vi "Administer Tables UI.vi"() -> ()   [LabVIEW 2019, in "LV-Data.PGSQL.lvclass"]
uses:
  LV-Data.PGSQL.lvclass
  Typedefs/Datatypes--enum.ctl
  <userlib>/_OpenG.lib/array/array.llb/Search 1D Array (String)__ogtk.vi
panel:
  in  "Safety":bool=TRUE
  in  "Delete Selected Table":bool
  in  "Delete Selected Column":bool
  in  "Rename Selected Table":bool
  in  "Update Selected Column Units":bool
  in  "Rename Selected Column":bool
  out "Path":string="llab_038:d001(TEST_TABLE--new_stuff(hippos))"
  out "selected table":string
  in  "New Column Units":string="discoveries"
  in  "New Column Name":string="successfulness"
  in  "Create New Column":bool
  in  "New Column Type":T1
  in  "Columns":i32(listbox)=-1
  in  "New Table Name":string="TEST_TABLE_2"
  in  "Create New Table":bool
  in  "Tables":i32(listbox)=-1
  in  "STOP":bool
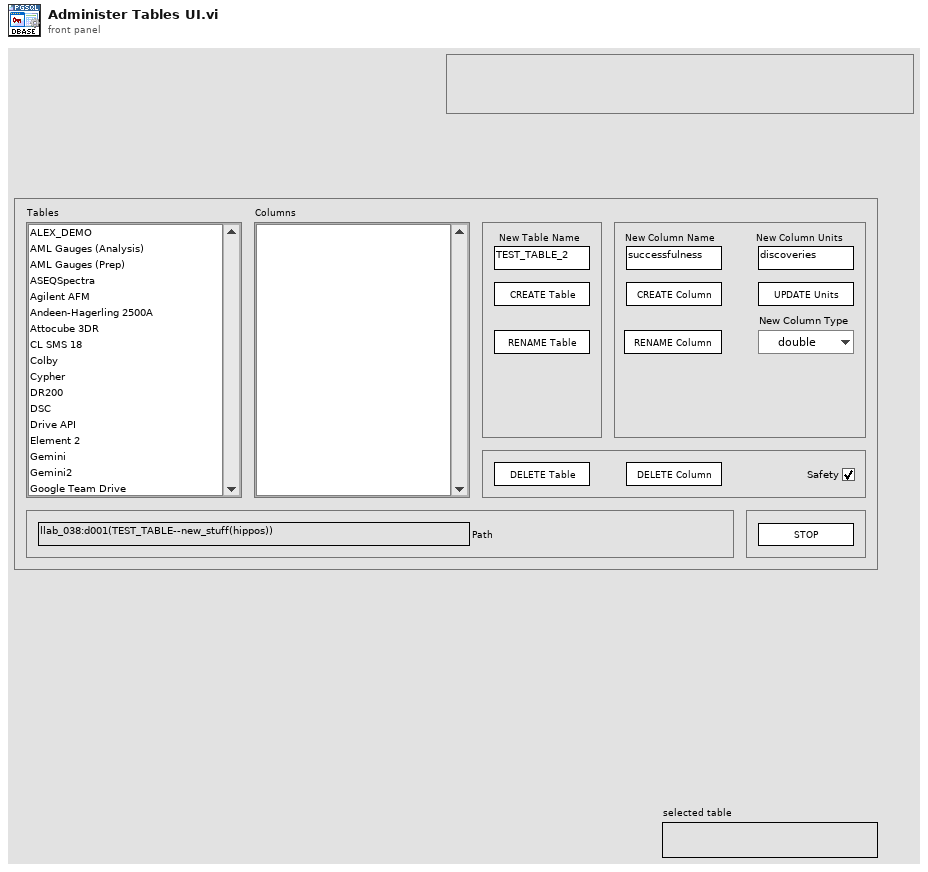
[diagram p1: front panel]
types:
  T1 = typedef "LV-Data.PGSQL.lvclass/Datatypes--enum.ctl" = enum16{"double", "string", "json", "integer", "boolean"}
  T2 = enum32{"Invalid", "Standard", "Closed", "Hidden", "Minimized", "Maximized"}
  T3 = enum32{"invalid app kind", "Development System", "Run Time System", "Student Edition", "Embedded LabVIEW", "Evaluation", "Custom"}
  T4 = cluster{"Core":cluster{"Current VI Reference":refnum<vi>, "Close Panel on Exit?":bool}, "Data.PG":refnum<class "LV-Data.PGSQL.lvclass">, "table names":string[], "table paths":string[], "column names":string[], "column units":string[], "column paths":string[], "new table name":string, "new column name":string, "new column data type":T1, "new column units":string, "selected table":string, "selected column":string, "selected table path":string, "selected column path":string, "selected column units":string}
  T5 = cluster{"Current VI Reference":refnum<vi>, "Close Panel on Exit?":bool}
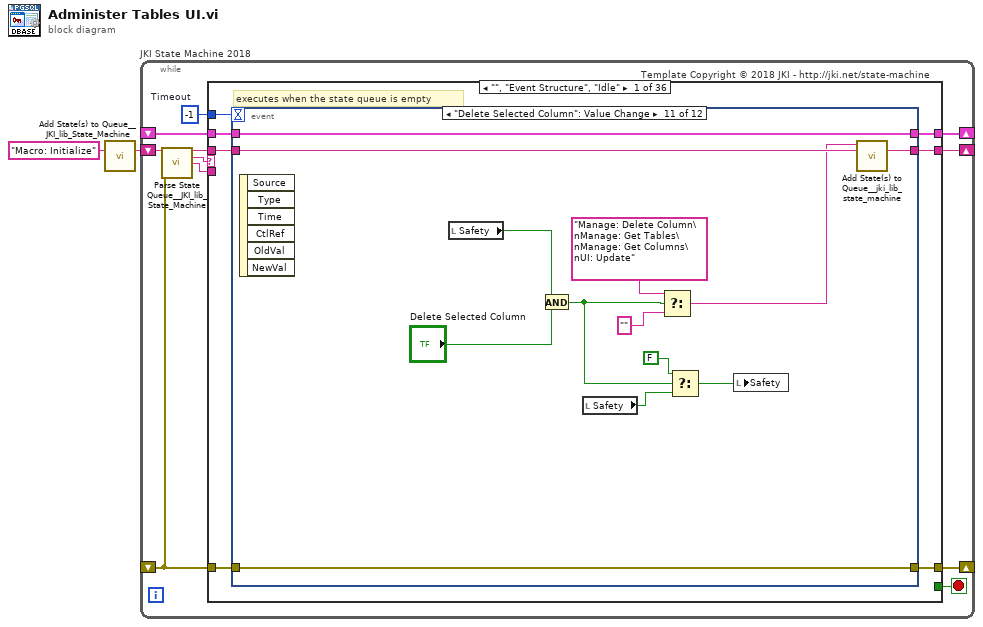
[diagram p0: block diagram]
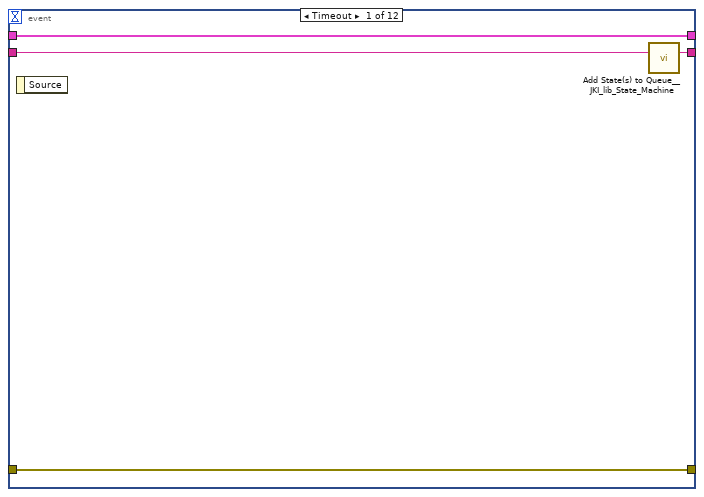
[diagram p2: hidden frame]
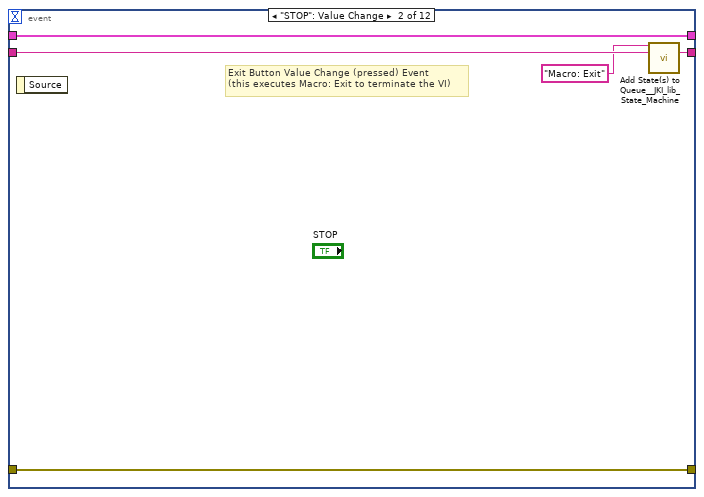
[diagram p3: hidden frame]
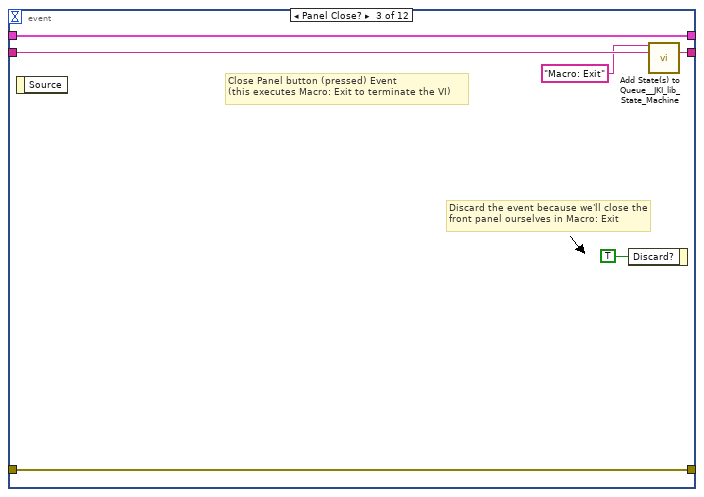
[diagram p4: hidden frame]
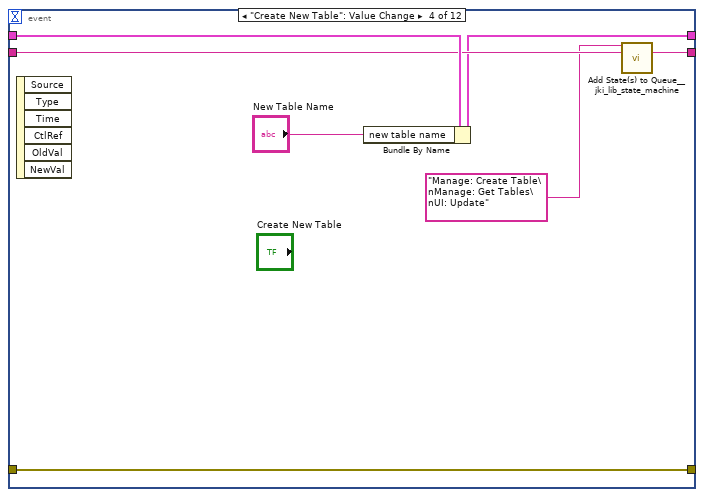
[diagram p5: hidden frame]
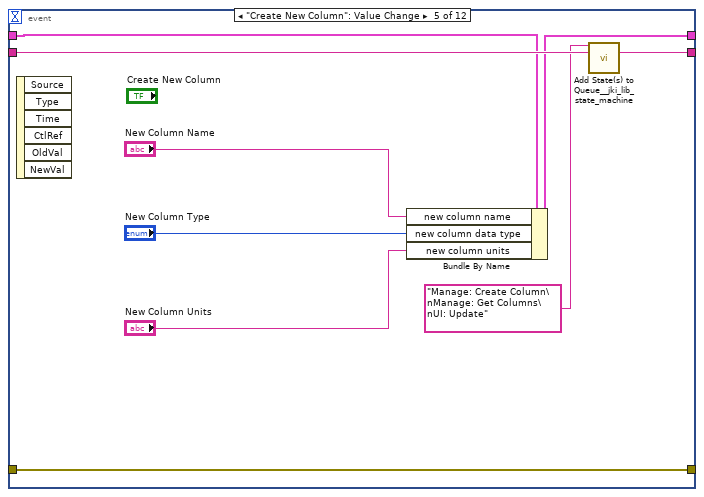
[diagram p6: hidden frame]
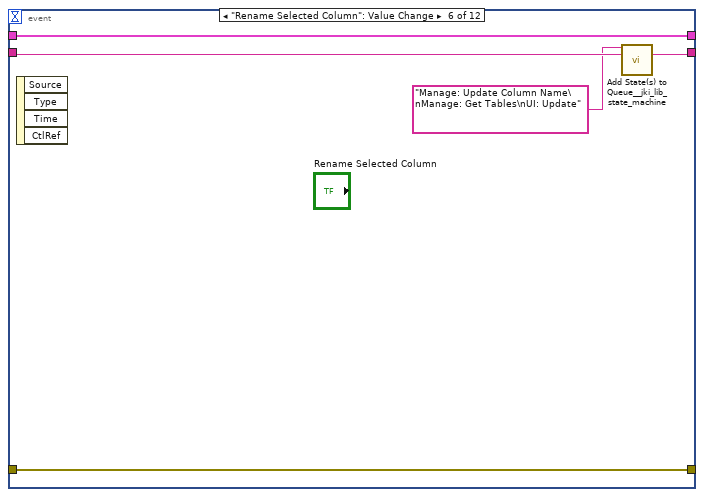
[diagram p7: hidden frame]
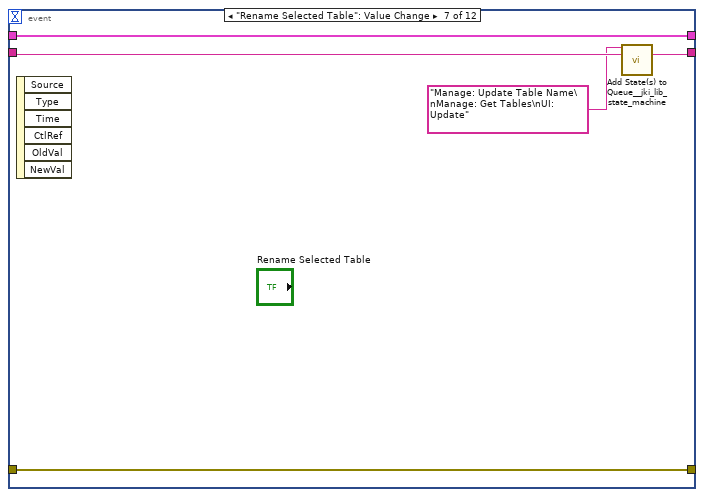
[diagram p8: hidden frame]
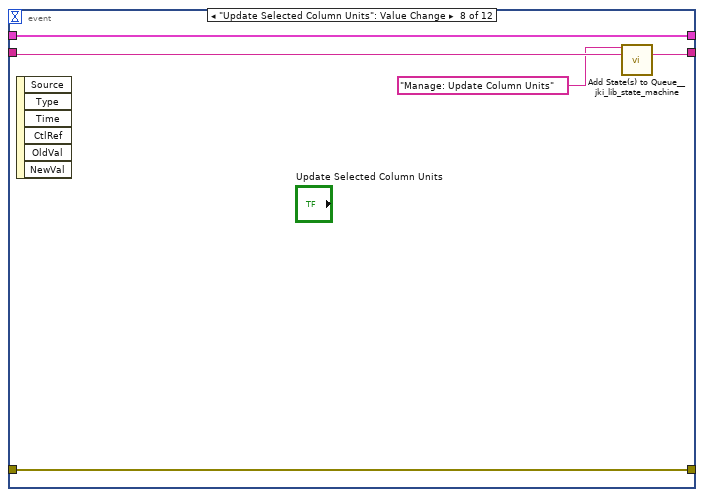
[diagram p9: hidden frame]
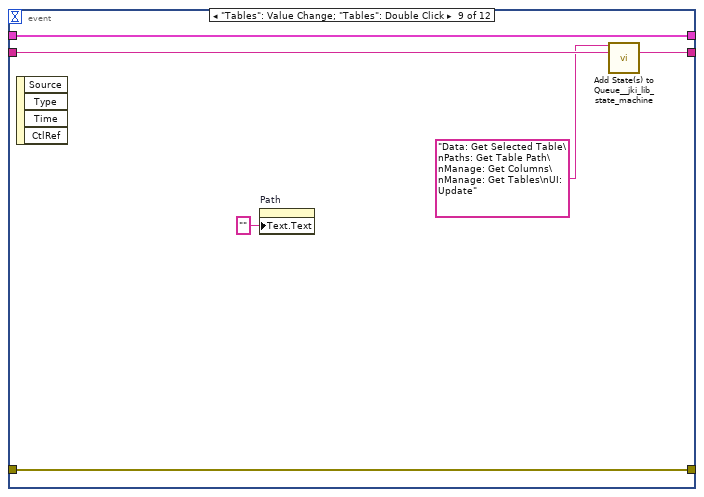
[diagram p10: hidden frame]
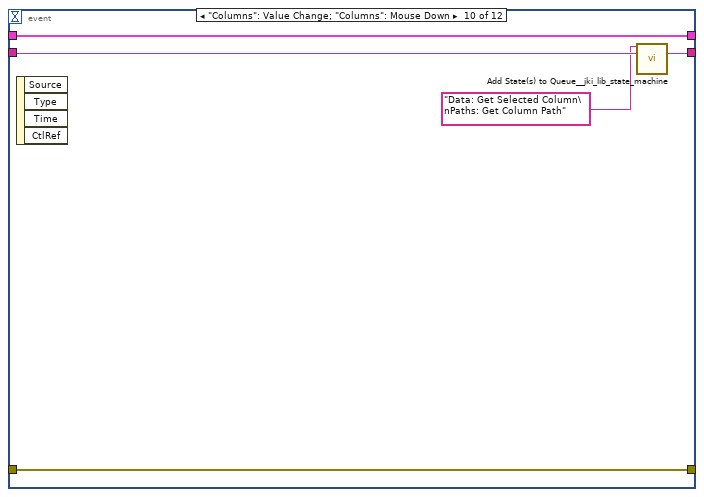
[diagram p11: hidden frame]
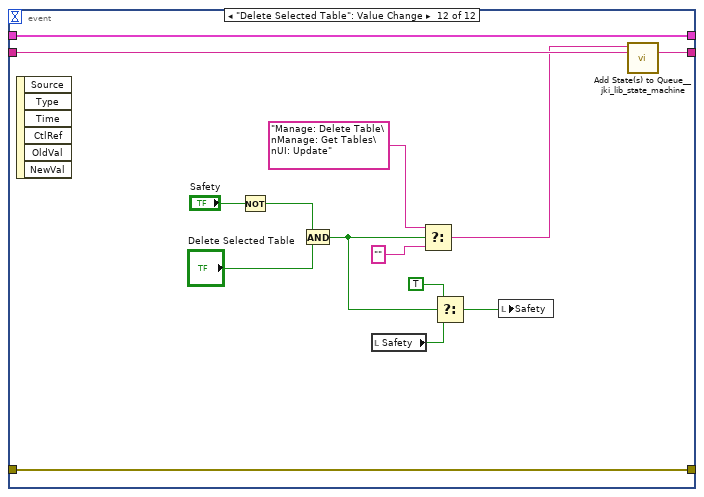
[diagram p12: hidden frame]
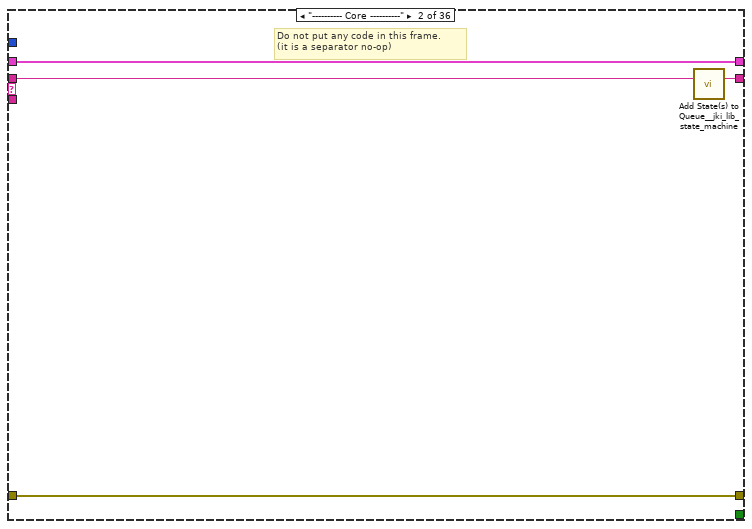
[diagram p13: hidden frame]
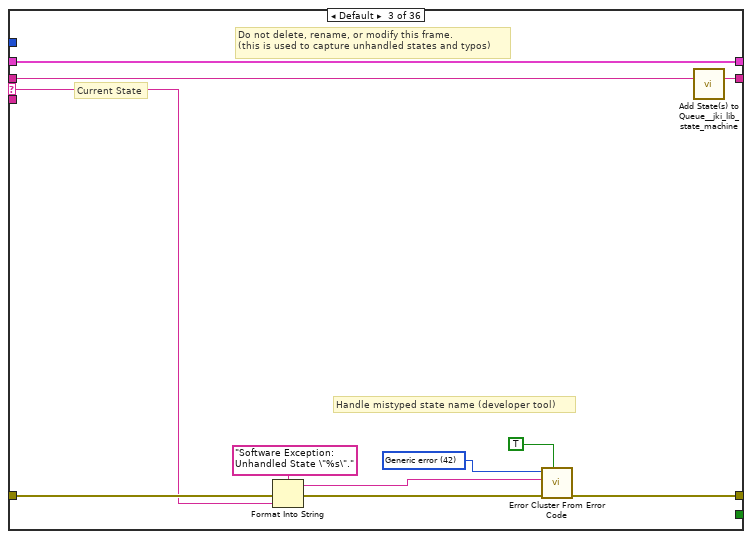
[diagram p14: hidden frame]
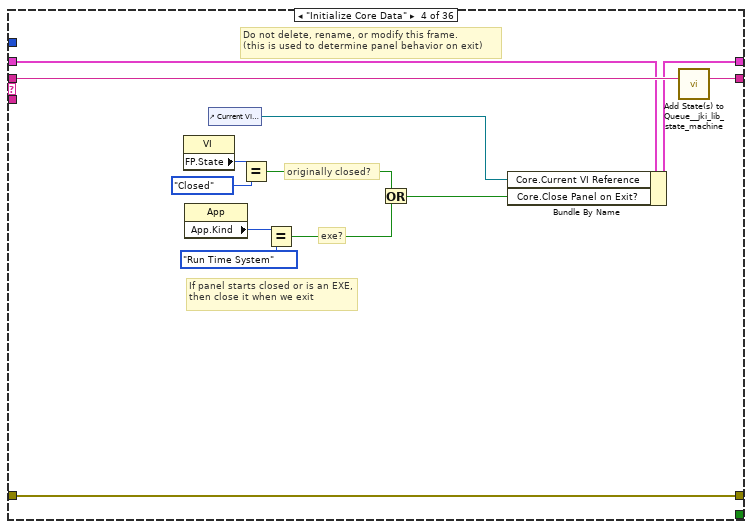
[diagram p15: hidden frame]
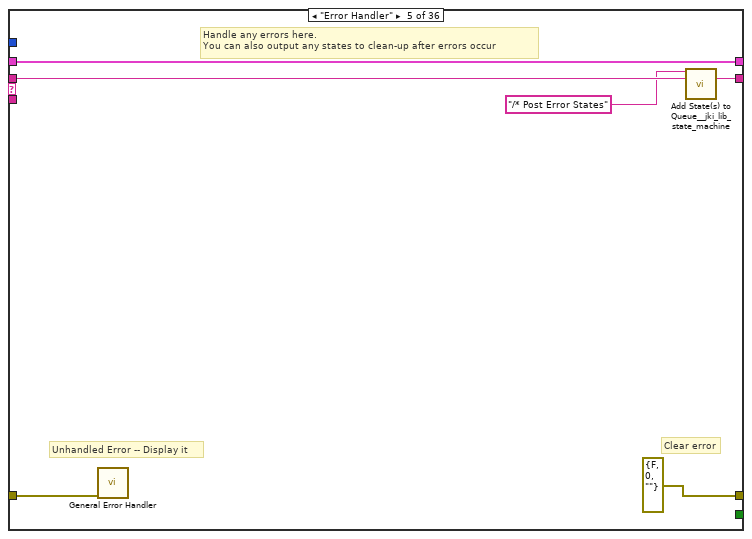
[diagram p16: hidden frame]
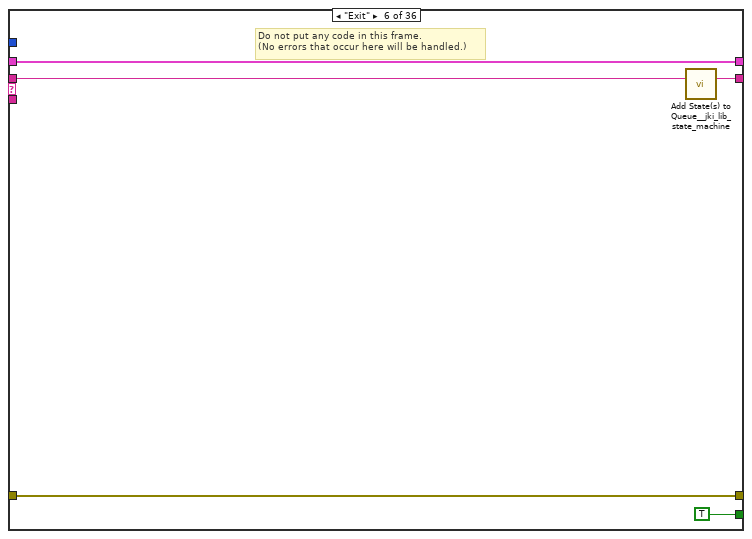
[diagram p17: hidden frame]
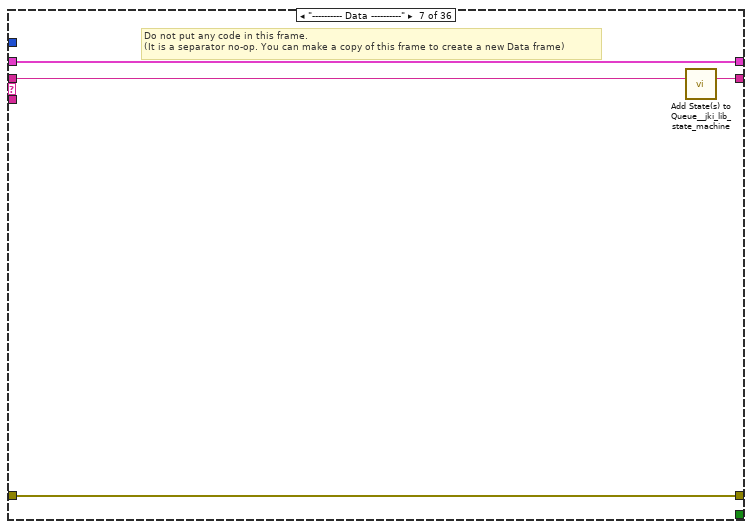
[diagram p18: hidden frame]
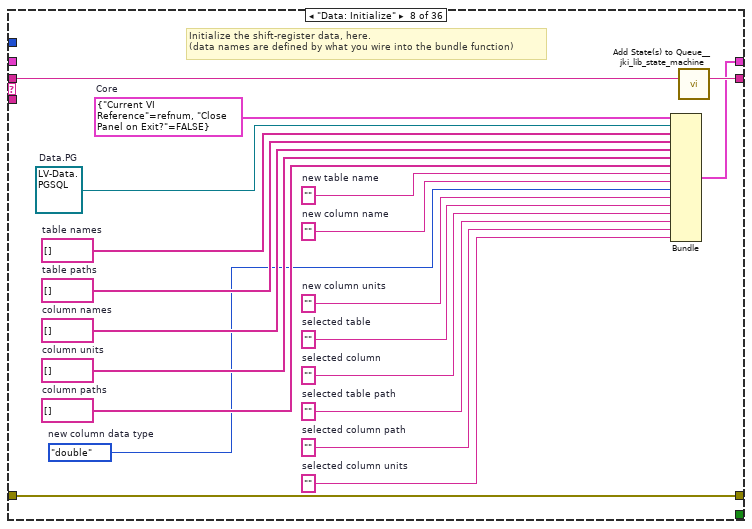
[diagram p19: hidden frame]
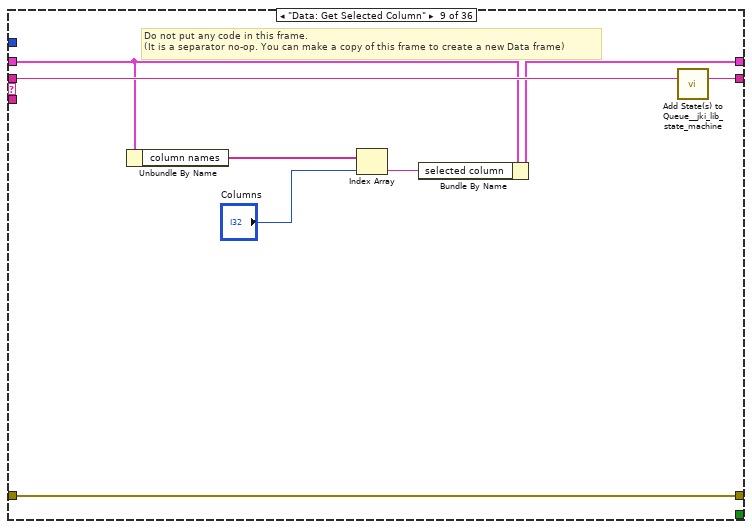
[diagram p20: hidden frame]
diagram:
  n1 = call <vilib>:"Add State(s) to Queue__JKI_lib_State_Machine.vi"("State(s) in (\"\")"="Macro: Initialize") -> ("States Out"=w2:string)  [unwired: 14 in]
  n2 = while "JKI State Machine 2018" {
    shift-right: [w6] -> _
    shift-left: _ -> [w5]
    shift-right: [w9] -> _
    shift-left: _ -> [w3]
    shift-right: [w8] -> _
    shift-left: w2 -> [w10]
    stop <- w7 stop-if-true
    w4 = -1  # Timeout
    # "Template Copyright © 2018 JKI - http://jki.net/state-machine"
    n3 = call <vilib>:"Parse State Queue__JKI_lib_State_Machine.vi"("State Queue"=w10, "Error In (no error)"=w3) -> ("Remaining States"=w12:string, "Current State"=w13:string, "Arguments"=w11:string)  [unwired: 11 in]
    n4 = case shown="\"\", \"Event Structure\", \"Idle\"" w13 {
      selector: w13 -> [_ _ w109 _ _ _ _ _ _ _ _ _ _ _ _ _ _ _ _ _ _ _ _ _ _ _ _ _ _ _ _ _ _ _ _ _]
      tunnel: w12 -> [w20 w108 w113 w132 w138 w143 w147 w167 w175 w183 w189 w193 w202 w210 w218 w224 w235 w304 w309 w319 w323 w332 w345 w356 w368 w378 w390 w400 w409 w418 w423 w431 w437 w441 w450 w462]
      tunnel: w11 -> [_ _ _ _ _ _ _ _ _ _ _ _ _ _ _ w219 w229 _ _ _ _ _ _ _ _ _ _ _ _ _ _ _ _ _ _ _]
      tunnel: w5 -> [w18 w105 w111 w125 w135 w141 w144 _ w168 w177 w184 w190 w194 w205 w215 w222 w231 w301 w306 w316 w320 w330 w343 w346 w359 w376 w380 w398 w402 w412 w420 w428 w435 w438 w448 w451]
      tunnel: [w17 w106 w115 w129 errorcluster {"status"=FALSE, "code"=0, "source"=""} ("error out") w140 w145 w165 w173 w181 w185 w191 w195 w208 w216 w220 w232 w302 w307 w317 w321 w325 w337 w348 w362 w373 w384 w392 w403 w413 w421 w424 w432 w439 w443 w453] -> w9
      tunnel: w3 -> [w16 w106 w114 w129 w134 w140 w145 w165 w173 w181 w186 w191 w200 w208 w216 w221 w233 w302 w307 w317 w321 w326 w338 w349 w365 w374 w385 w394 w404 w414 w421 w425 w433 w439 w444 w456]
      tunnel: [w19 w107 w112 w131 w137 w142 w146 w166 w174 w182 w188 w192 w201 w209 w217 w223 w234 w303 w308 w318 w322 w331 w344 w355 w367 w377 w389 w399 w410 w419 w422 w430 w436 w440 w449 w463] -> w8
      tunnel: [_ _ _ _ _ TRUE _ _ _ _ _ _ _ _ _ _ _ _ _ _ _ _ _ _ _ _ _ _ _ _ _ _ _ _ _ _] -> w7
      tunnel: [w15 w105 w111 w130 w135 w141 w144 w150 w170 w178 w184 w190 w194 w205 w215 w222 w231 w301 w306 w316 w320 w329 w342 w352 w361 w375 w383 w398 w401 w411 w420 w429 w435 w438 w447 w464] -> w6
      tunnel: w4 -> [w14 _ _ _ _ _ _ _ _ _ _ _ _ _ _ _ _ _ _ _ _ _ _ _ _ _ _ _ _ _ _ _ _ _ _ _]
      frame "", "Event Structure", "Idle" {
        # "executes when the state queue is empty"
        n5 = event shown="[10] \"Delete Selected Column\": Value Change" {
          selector: _ -> [_ _ _ _ _ _ _ _ _ _ _ _]
          dyn-events: _ -> [_ _ _ _ _ _ _ _ _ _ _ _]
          timeout: w14 -> [_ _ _ _ _ _ _ _ _ _ _ _]
          tunnel: w20 -> [w24 w29 w35 w39 w47 w54 w59 w64 w70 w75 w87 w103]
          tunnel: [w23 w28 w34 w38 w48 w55 w60 w65 w71 w76 w89 w104] -> w19
          tunnel: w18 -> [w21 w26 w32 w41 w46 w53 w58 w63 w67 w77 w90 w102]
          tunnel: [w22 w27 w33 w42 w49 w56 w61 w66 w72 w73 w88 w101] -> w17
          tunnel: w16 -> [w22 w27 w33 w42 w49 w56 w61 w66 w72 w73 w88 w101]
          tunnel: [w21 w26 w32 w36 w45 w53 w58 w63 w67 w77 w90 w102] -> w15
          event Timeout {
            n6 = event-data() -> ()  [unwired: 1 in, 1 out]
            n7 = call <vilib>:"Add State(s) to Queue__JKI_lib_State_Machine.vi"("State(s) in (\"\")"=w24) -> ("States Out"=w23:string)  [unwired: 14 in]
          }
          event "STOP": Value Change {
            # "Exit Button Value Change (pressed) Event\n(this executes Macro: Exit to terminate the VI)"
            n8 = event-data() -> ()  [unwired: 1 in, 1 out]
            n9 = call <vilib>:"Add State(s) to Queue__JKI_lib_State_Machine.vi"("State(s) in Front (\"\")"="Macro: Exit", "State(s) in (\"\")"=w29) -> ("States Out"=w28:string)  [unwired: 13 in]
          }
          event Panel Close? {
            # "Discard the event because we'll close the front panel ourselves in Macro: Exit"
            # "Close Panel button (pressed) Event\n(this executes Macro: Exit to terminate the VI)"
            n10 = event-data() -> ()  [unwired: 1 in, 1 out]
            n11 = event-data("Discard?"=TRUE) -> ()  [unwired: 1 in, 1 out]
            n12 = call <vilib>:"Add State(s) to Queue__JKI_lib_State_Machine.vi"("State(s) in Front (\"\")"="Macro: Exit", "State(s) in (\"\")"=w35) -> ("States Out"=w34:string)  [unwired: 13 in]
          }
          event "Create New Table": Value Change {
            n13 = event-data() -> ()  [unwired: 1 in, 6 out]
            n14 = Bundle By Name(cluster=w41, "new table name"="New Table Name") -> (w36:T4)
            n15 = call <vilib>:"Add State(s) to Queue__jki_lib_state_machine.vi"("State(s) in Front (\"\")"="Manage: Create Table\nManage: Get Tables\nUI: Update" ("State(s) in Front (\"\")"), "State(s) in (\"\")"=w39) -> ("States Out"=w38:string)  [unwired: 13 in]
          }
          event "Create New Column": Value Change {
            n16 = event-data() -> ()  [unwired: 1 in, 6 out]
            n17 = Bundle By Name(cluster=w46, "new column name"="New Column Name", "new column data type"="New Column Type", "new column units"="New Column Units") -> (w45:T4)
            n18 = call <vilib>:"Add State(s) to Queue__jki_lib_state_machine.vi"("State(s) in Front (\"\")"="Manage: Create Column\nManage: Get Columns\nUI: Update" ("State(s) in Front (\"\")"), "State(s) in (\"\")"=w47) -> ("States Out"=w48:string)  [unwired: 13 in]
          }
          event "Rename Selected Column": Value Change {
            n19 = event-data() -> ()  [unwired: 1 in, 4 out]
            n20 = call <vilib>:"Add State(s) to Queue__jki_lib_state_machine.vi"("State(s) in Front (\"\")"="Manage: Update Column Name\nManage: Get Tables\nUI: Update" ("State(s) in Front (\"\")"), "State(s) in (\"\")"=w54) -> ("States Out"=w55:string)  [unwired: 13 in]
          }
          event "Rename Selected Table": Value Change {
            n21 = event-data() -> ()  [unwired: 1 in, 6 out]
            n22 = call <vilib>:"Add State(s) to Queue__jki_lib_state_machine.vi"("State(s) in Front (\"\")"="Manage: Update Table Name\nManage: Get Tables\nUI: Update" ("State(s) in Front (\"\")"), "State(s) in (\"\")"=w59) -> ("States Out"=w60:string)  [unwired: 13 in]
          }
          event "Update Selected Column Units": Value Change {
            n23 = event-data() -> ()  [unwired: 1 in, 6 out]
            n24 = call <vilib>:"Add State(s) to Queue__jki_lib_state_machine.vi"("State(s) in Front (\"\")"="Manage: Update Column Units" ("State(s) in Front (\"\")"), "State(s) in (\"\")"=w64) -> ("States Out"=w65:string)  [unwired: 13 in]
          }
          event "Tables": Value Change; "Tables": Double Click {
            n25 = event-data() -> ()  [unwired: 1 in, 4 out]
            n26 = property on="Path" class="Str"("Text.Text"="") -> ()  [unwired: 2 in, 2 out]
            n27 = call <vilib>:"Add State(s) to Queue__jki_lib_state_machine.vi"("State(s) in Front (\"\")"="Data: Get Selected Table\nPaths: Get Table Path\nManage: Get Columns\nManage: Get Tables\nUI: Update" ("State(s) in Front (\"\")"), "State(s) in (\"\")"=w70) -> ("States Out"=w71:string)  [unwired: 13 in]
          }
          event "Columns": Value Change; "Columns": Mouse Down {
            n28 = event-data() -> ()  [unwired: 1 in, 4 out]
            n29 = call <vilib>:"Add State(s) to Queue__jki_lib_state_machine.vi"("State(s) in Front (\"\")"="Data: Get Selected Column\nPaths: Get Column Path", "State(s) in (\"\")"=w75) -> ("States Out"=w76:string)  [unwired: 13 in]
          }
          event "Delete Selected Column": Value Change {
            n30 = event-data() -> ()  [unwired: 1 in, 6 out]
            n31 = local read "Safety"() -> (w79:bool)
            n32 = And(x=w79, y="Delete Selected Column") -> (x .and. y?=w81:bool)
            n33 = local read "Safety"() -> (w82:bool)
            n34 = Select(t="Manage: Delete Column\nManage: Get Tables\nManage: Get Columns\nUI: Update" ("State(s) in Front (\"\")"), s=w81, f="") -> (s? t:f=w84:string)
            n35 = Select(t=FALSE, s=w81, f=w82) -> (s? t:f=w83:bool)
            n36 = local write "Safety"(w83) -> ()
            n37 = call <vilib>:"Add State(s) to Queue__jki_lib_state_machine.vi"("State(s) in Front (\"\")"=w84, "State(s) in (\"\")"=w87) -> ("States Out"=w89:string)  [unwired: 13 in]
          }
          event "Delete Selected Table": Value Change {
            n38 = event-data() -> ()  [unwired: 1 in, 6 out]
            n39 = Not(x="Safety") -> (.not. x?=w92:bool)
            n40 = And(x=w92, y="Delete Selected Table") -> (x .and. y?=w94:bool)
            n41 = local read "Safety"() -> (w91:bool)
            n42 = Select(t="Manage: Delete Table\nManage: Get Tables\nUI: Update" ("State(s) in Front (\"\")"), s=w94, f="") -> (s? t:f=w96:string)
            n43 = Select(t=TRUE, s=w94, f=w91) -> (s? t:f=w95:bool)
            n44 = local write "Safety"(w95) -> ()
            n45 = call <vilib>:"Add State(s) to Queue__jki_lib_state_machine.vi"("State(s) in Front (\"\")"=w96, "State(s) in (\"\")"=w103) -> ("States Out"=w104:string)  [unwired: 13 in]
          }
        }
      }
      frame "---------- Core ----------" {
        # "Do not put any code in this frame.\n(it is a separator no-op)"
        n46 = call <vilib>:"Add State(s) to Queue__jki_lib_state_machine.vi"("State(s) in (\"\")"=w108) -> ("States Out"=w107:string)  [unwired: 14 in]
      }
      frame Default {
        w118 = 42 items=["No error", "Argument error", "Memory is full", "Out of zone", "End of file", "File already open", "Generic file I/O error", "File not found", "File permission error", "Disk is full", "Duplicate path", "Too many files open", "System feature not enabled", "Resource file not found", "Cannot add resource", "Resource not found", "Image not found", "Image memory error", "Pen does not exist", "Config type invalid", "Config token not found", "Config parse error", "Config memory error", "Bad external code format", "Bad external code offset", "External code not present", "Null window", "Destroy window error", "Null menu", "Print aborted", "Bad print record", "Print driver error", "Windows error during printing", "Memory error during printing", "Print dialog error", "Generic print error", "Invalid device refnum", "Device not found", "Device parameter error", "Device unit error", "Cannot open device", "Device call aborted", "Generic error", "Cancelled by user", "Object ID too low", "Object ID too high", "Object not in heap", "Unknown heap", "Unknown object (invalid DefProc)", "Unknown object (DefProc not in table)", "Message out of range", "Invalid (null) method", "Unknown message", "Manager call not supported", "Bad address", "Network operation in progress", "Network operation timed out", "Connection is busy", "Network attribute not supported", "Network error", "Address in use", "System out of memory", "Connection aborted", "Connection refused", "Not connected", "Already connected", "Connection closed", "Initialization error (interapplication manager)", "Bad occurrence", "Wait on unbound occurrence handler", "Occurrence queue overflow", "Datalog type conflict", "Unused", "Unrecognized type (interapplication manager)", "Memory corrupt", "Failed to make temporary DLL", "Old CIN version", "Drag socket not found", "Failed to load drop-object", "Failed to register OLE object", "Failed to release OLE object", "Format specifier type mismatch", "Unknown format specifier", "Too few format specifiers", "Too many format specifiers", "Scan failed", "Newer CIN version", "Error converting to variant", "Runtime menu error", "Password tampered", "Variant attribute not found", "Incompatible variant data type", "Event data is not available", "Event Store is not present", "Occurrence is not found", "Event Queue is not created", "Event info is not available", "Refnum passed is NULL", "Error retrieving Class GUID", "Error retrieving CoClass GUID", "Error retrieving TypeLib GUID.", "Bad built application magic bytes.", "Specific driver is different from the specific driver associated with the Logical Name.", "There is no session opened to the class driver.", "Max Error", "MAX - Error with config objects", "MAX - Error loading configuration", "MAX - Group not supported"]
        # "Current State"
        # "Do not delete, rename, or modify this frame.\n(this is used to capture unhandled states and typos)"
        # "Handle mistyped state name (developer tool)"
        n47 = Format Into String(format string="Software Exception: Unhandled State \"%s\"." ("message"), error in=w114, w109) -> (resulting string=w117:string, error out=w116:errorcluster)  [unwired: 1 in]
        n48 = call <vilib>:"Error Cluster From Error Code.vi"("show call chain? (False)"=TRUE, "error in (no error)"=w116, "error message (\"\")"=w117, "error code (0)"=w118) -> ("error out"=w115:errorcluster)  [unwired: 5 in]
        n49 = call <vilib>:"Add State(s) to Queue__jki_lib_state_machine.vi"("State(s) in (\"\")"=w113) -> ("States Out"=w112:string)  [unwired: 14 in]
      }
      frame "Initialize Core Data" {
        # "Do not delete, rename, or modify this frame.\n(this is used to determine panel behavior on exit)"
        # "originally closed?"
        # "exe?"
        # "If panel starts closed or is an EXE, then close it when we exit"
        n50 = property class="VI"() -> ("FP.State"=w122:T2)  [unwired: 2 in, 2 out]
        n51 = property class="App"() -> ("App.Kind"=w128:T3)  [unwired: 2 in, 2 out]
        n52 = control-ref of="Current VI Reference"() -> (w123:refnum<vi>)
        n53 = Equal?(x=w122, y=T2."Closed" ("Front Panel Window:State")) -> (x = y?=w120:bool)
        n54 = Equal?(x=w128, y=T3."Run Time System" ("Application:Kind")) -> (x = y?=w126:bool)
        n55 = Or(x=w120, y=w126) -> (x .or. y?=w124:bool)
        n56 = Bundle By Name(cluster=w125, "Core.Current VI Reference"=w123, "Core.Close Panel on Exit?"=w124) -> (w130:T4)
        n57 = call <vilib>:"Add State(s) to Queue__jki_lib_state_machine.vi"("State(s) in (\"\")"=w132) -> ("States Out"=w131:string)  [unwired: 14 in]
      }
      frame "Error Handler" {
        # "Unhandled Error -- Display it"
        # "Handle any errors here.\nYou can also output any states to clean-up after errors occur"
        # "Clear error"
        n58 = call <vilib>:"General Error Handler.vi"("error in (no error)"=w134) -> ()  [unwired: 10 in, 5 out]
        n59 = call <vilib>:"Add State(s) to Queue__jki_lib_state_machine.vi"("State(s) in Front (\"\")"="/* Post Error States", "State(s) in (\"\")"=w138) -> ("States Out"=w137:string)  [unwired: 13 in]
      }
      frame "Exit" {
        # "Do not put any code in this frame.\n(No errors that occur here will be handled.)"
        n60 = call <vilib>:"Add State(s) to Queue__jki_lib_state_machine.vi"("State(s) in (\"\")"=w143) -> ("States Out"=w142:string)  [unwired: 14 in]
      }
      frame "---------- Data ----------" {
        # "Do not put any code in this frame.\n(It is a separator no-op. You can make a copy of this frame to create a new Data frame)"
        n61 = call <vilib>:"Add State(s) to Queue__jki_lib_state_machine.vi"("State(s) in (\"\")"=w147) -> ("States Out"=w146:string)  [unwired: 14 in]
      }
      frame "Data: Initialize" {
        w148 = Datatypes--enum."double"  # new column data type
        w151 = ""  # selected column units
        w152 = ""  # selected column path
        w153 = ""  # selected table path
        w154 = ""  # selected column
        w155 = ""  # selected table
        w156 = ""  # new column units
        w157 = ""  # new column name
        w158 = ""  # new table name
        w159 = string[] []  # column paths
        w160 = string[] []  # column units
        w161 = string[] []  # column names
        w162 = string[] []  # table paths
        w163 = string[] []  # table names
        w149 = refnum<class "LV-Data.PGSQL.lvclass"> refnum  # Data.PG
        w164 = T5 {"Current VI Reference"=refnum, "Close Panel on Exit?"=FALSE}  # Core
        # "Initialize the shift-register data, here.\n(data names are defined by what you wire into the bundle function)"
        n62 = Bundle("Core"=w164, "Data.PG"=w149, "table names"=w163, "table paths"=w162, "column names"=w161, "column units"=w160, "column paths"=w159, "new table name"=w158, "new column name"=w157, "new column data type"=w148, "new column units"=w156, "selected table"=w155, "selected column"=w154, "selected table path"=w153, "selected column path"=w152, "selected column units"=w151) -> (w150:T4)  [unwired: 1 in]
        n63 = call <vilib>:"Add State(s) to Queue__jki_lib_state_machine.vi"("State(s) in (\"\")"=w167) -> ("States Out"=w166:string)  [unwired: 14 in]
      }
      frame "Data: Get Selected Column" {
        # "Do not put any code in this frame.\n(It is a separator no-op. You can make a copy of this frame to create a new Data frame)"
        n64 = Unbundle By Name(w168) -> ("column names"=w171:string[])
        n65 = Index Array(array=w171, index="Columns") -> (element=w169:string)
        n66 = Bundle By Name(cluster=w168, "selected column"=w169) -> (w170:T4)
        n67 = call <vilib>:"Add State(s) to Queue__jki_lib_state_machine.vi"("State(s) in (\"\")"=w175) -> ("States Out"=w174:string)  [unwired: 14 in]
      }
      frame "Data: Get Selected Table" {
        # "Do not put any code in this frame.\n(It is a separator no-op. You can make a copy of this frame to create a new Data frame)"
        n68 = Unbundle By Name(w177) -> ("table names"=w179:string[])
        n69 = Index Array(array=w179, index="Tables") -> (element=w180:string)
        n70 = Bundle By Name(cluster=w177, "selected table"=w180) -> (w178:T4)
        n71 = call <vilib>:"Add State(s) to Queue__jki_lib_state_machine.vi"("State(s) in (\"\")"=w183) -> ("States Out"=w182:string)  [unwired: 14 in]
      }
      frame "Data: Cleanup" {
        # "Cleanup any data and references, here.\n(this is called automatically, by the Macro: Exit)"
        n72 = Unbundle By Name(w184) -> ("Core.Current VI Reference"=w187:refnum<vi>)
        n73 = Close Reference(reference=w187, error in (no error)=w186) -> (error out=w185:errorcluster)
        n74 = call <vilib>:"Add State(s) to Queue__jki_lib_state_machine.vi"("State(s) in (\"\")"=w189) -> ("States Out"=w188:string)  [unwired: 14 in]
      }
      frame "---------- UI ----------" {
        # "Do not put any code in this frame.\n(It is a separator no-op. You can make a copy of this frame to create a new UI frame)"
        n75 = call <vilib>:"Add State(s) to Queue__jki_lib_state_machine.vi"("State(s) in (\"\")"=w193) -> ("States Out"=w192:string)  [unwired: 14 in]
      }
      frame "UI: Initialize" {
        # "Initialize the User Interface, here.\n(this is called automatically, by the Macro: Init)"
        n76 = Unbundle By Name(w194) -> ("table names"=w199:string[], "column names"=w198:string[], "selected table"=→"selected table":string)
        n77 = property on="Tables" class="LstBox (strict)"("Item Names"=w199) -> ()  [unwired: 2 in, 2 out]
        n78 = property on="Columns" class="LstBox (strict)"("Item Names"=w198) -> ()  [unwired: 2 in, 2 out]
        n79 = property on="Path" class="Str"("Text.Text"="") -> ()  [unwired: 2 in, 2 out]
        n80 = call <userlib>:"Fit VI window to Largest Dec__ogtk.vi"("error in (no error)"=w200) -> ("error out"=w195:errorcluster)  [unwired: 5 in, 1 out]
        n81 = call <vilib>:"Add State(s) to Queue__jki_lib_state_machine.vi"("State(s) in (\"\")"=w202) -> ("States Out"=w201:string)  [unwired: 14 in]
      }
      frame "UI: Update" {
        # "Initialize the User Interface, here.\n(this is called automatically, by the Macro: Init)"
        n82 = Unbundle By Name(w205) -> ("table names"=w207:string[], "column names"=w206:string[], "selected table"=w204:string, "selected column path"=w203:string)
        n83 = property on="Tables" class="LstBox (strict)"("Item Names"=w207) -> ()  [unwired: 2 in, 2 out]
        n84 = local write "selected table"(w204) -> ()
        n85 = property on="Columns" class="LstBox (strict)"("Item Names"=w206) -> ()  [unwired: 2 in, 2 out]
        n86 = property on="Path" class="Str"("Text.Text"=w203) -> ()  [unwired: 2 in, 2 out]
        n87 = call <vilib>:"Add State(s) to Queue__jki_lib_state_machine.vi"("State(s) in (\"\")"=w210) -> ("States Out"=w209:string)  [unwired: 14 in]
      }
      frame "UI: Choose Column" {
        # "Do not put any code in this frame.\n(It is a separator no-op. You can make a copy of this frame to create a new UI frame)"
        n88 = Unbundle By Name(w215) -> ("column names"=w214:string[], "selected column"=w213:string)
        n89 = call-poly <userlib>:"Search Array__ogtk.vi"("Array"=w214, "Element Data"=w213) -> ("Indices of Elements"=w212:i32[])  [unwired: 7 in]
        n90 = Index Array(array=w212) -> (element=w211:i32)  [unwired: 1 in]
        n91 = property on="Columns" class="LstBox (strict)"("Value"=w211) -> ()  [unwired: 2 in, 2 out]
        n92 = call <vilib>:"Add State(s) to Queue__jki_lib_state_machine.vi"("State(s) in (\"\")"=w218) -> ("States Out"=w217:string)  [unwired: 14 in]
      }
      frame "UI: Cursor Set" {
        # "Argument"
        # "Set and Unset Cursor Busy.\n(Usage: \"UI: Cursor Set >> Busy|Idle\")"
        n93 = case shown="\"Idle\", Default" w219 {
          tunnel: w221 -> [w226 w228]
          tunnel: [w225 w227] -> w220
          frame "Idle", Default {
            n94 = call <vilib>:"Unset Busy.vi"("error in (no error)"=w226) -> ("error out"=w225:errorcluster)  [unwired: 10 in]
          }
          frame "Busy" {
            n95 = call <vilib>:"Set Busy.vi"("error in (no error)"=w228) -> ("error out"=w227:errorcluster)  [unwired: 9 in, 1 out]
          }
        }
        n96 = call <vilib>:"Add State(s) to Queue__jki_lib_state_machine.vi"("State(s) in (\"\")"=w224) -> ("States Out"=w223:string)  [unwired: 14 in]
      }
      frame "UI: Front Panel State" {
        # "Argument"
        # "Set Front Panel Open or Closed\n(Usage: \"UI: Front Panel State >> Open|Close\")"
        n97 = Unbundle By Name(w231) -> ("Core.Current VI Reference"=w230:refnum<vi>)
        n98 = case shown="\"Open\", \"Standard\", Default" w229 {
          tunnel: w233 -> [w241 w256 w267 w280 w293]
          tunnel: [w243 w257 w269 w282 w295] -> w232
          tunnel: w230 -> [w242 w254 w268 w281 w294]
          frame "Open", "Standard", Default {
            w236 = T2."Standard" ("State")
            n99 = property class="VI"(reference=w242, error in=w241) -> (reference out=w239:refnum<vi>, error out=w240:errorcluster, "FP.State"=w238:T2)
            n100 = Not Equal?(x=w238, y=w236) -> (x != y?=w237:bool)
            n101 = case shown="False" w237 {
              tunnel: [w247 w249] -> w243
              tunnel: w240 -> [w246 w249]
              tunnel: w239 -> [w245 _]
              tunnel: w236 -> [w244 _]
              frame True {
                n102 = invoke class="VI" method="FP.Open"(reference=w245, error in=w246, "Activate"=TRUE, "State"=w244) -> (error out=w247:errorcluster)  [unwired: 1 in, 4 out]
              }
              frame False {
              }
            }
          }
          frame "Close", "Closed" {
            n103 = property class="VI"(reference=w254, error in=w256) -> (reference out=w253:refnum<vi>, error out=w255:errorcluster, "FP.State"=w251:T2)
            n104 = Not Equal?(x=w251, y=T2."Closed" ("Front Panel Window:State")) -> (x != y?=w250:bool)
            n105 = case shown="True" w250 {
              tunnel: [w258 w261] -> w257
              tunnel: w255 -> [w258 w260]
              tunnel: w253 -> [_ w259]
              frame False {
              }
              frame True {
                n106 = invoke class="VI" method="FP.Close"(reference=w259, error in=w260) -> (error out=w261:errorcluster)  [unwired: 1 in, 2 out]
              }
            }
          }
          frame "Hidden", "Hide" {
            w262 = T2."Hidden" ("State")
            n107 = property class="VI"(reference=w268, error in=w267) -> (reference out=w265:refnum<vi>, error out=w266:errorcluster, "FP.State"=w264:T2)
            n108 = Not Equal?(x=w264, y=w262) -> (x != y?=w263:bool)
            n109 = case shown="True" w263 {
              tunnel: [w273 w274] -> w269
              tunnel: w266 -> [w272 w274]
              tunnel: w265 -> [w271 _]
              tunnel: w262 -> [w270 _]
              frame True {
                n110 = invoke class="VI" method="FP.Open"(reference=w271, error in=w272, "State"=w270) -> (error out=w273:errorcluster)  [unwired: 2 in, 4 out]
              }
              frame False {
              }
            }
          }
          frame "Minimize", "Minimized" {
            w275 = T2."Minimized" ("State")
            n111 = property class="VI"(reference=w281, error in=w280) -> (reference out=w278:refnum<vi>, error out=w279:errorcluster, "FP.State"=w277:T2)
            n112 = Not Equal?(x=w277, y=w275) -> (x != y?=w276:bool)
            n113 = case shown="True" w276 {
              tunnel: [w286 w287] -> w282
              tunnel: w279 -> [w285 w287]
              tunnel: w278 -> [w284 _]
              tunnel: w275 -> [w283 _]
              frame True {
                n114 = invoke class="VI" method="FP.Open"(reference=w284, error in=w285, "State"=w283) -> (error out=w286:errorcluster)  [unwired: 2 in, 4 out]
              }
              frame False {
              }
            }
          }
          frame "Maximize", "Maximized" {
            w288 = T2."Maximized" ("State")
            n115 = property class="VI"(reference=w294, error in=w293) -> (reference out=w291:refnum<vi>, error out=w292:errorcluster, "FP.State"=w290:T2)
            n116 = Not Equal?(x=w290, y=w288) -> (x != y?=w289:bool)
            n117 = case shown="True" w289 {
              tunnel: [w299 w300] -> w295
              tunnel: w292 -> [w298 w300]
              tunnel: w291 -> [w297 _]
              tunnel: w288 -> [w296 _]
              frame True {
                n118 = invoke class="VI" method="FP.Open"(reference=w297, error in=w298, "State"=w296) -> (error out=w299:errorcluster)  [unwired: 2 in, 4 out]
              }
              frame False {
              }
            }
          }
        }
        n119 = call <vilib>:"Add State(s) to Queue__jki_lib_state_machine.vi"("State(s) in (\"\")"=w235) -> ("States Out"=w234:string)  [unwired: 14 in]
      }
      frame "---------- Macro ----------" {
        # "Do not put any code in this frame.\n(It is a separator no-op. You can make a copy of this frame to create a new Macro frame)"
        n120 = call <vilib>:"Add State(s) to Queue__jki_lib_state_machine.vi"("State(s) in (\"\")"=w304) -> ("States Out"=w303:string)  [unwired: 14 in]
      }
      frame "Macro: Initialize" {
        # "Initialization Macro\n(This is called once, when the VI starts)"
        n121 = call <vilib>:"Add State(s) to Queue__jki_lib_state_machine.vi"("State(s) in Front (\"\")"="Data: Initialize\nInitialize Core Data\nUI: Initialize\nUI: Front Panel State >> Open\n\nConnection: Open\nManage: Get Tables\nUI: Update", "State(s) in (\"\")"=w309) -> ("States Out"=w308:string)  [unwired: 13 in]
      }
      frame "Macro: Exit" {
        # "Exit Macro\n(This is called once, when the VI exits)"
        n122 = Unbundle By Name(w316) -> ("Core.Close Panel on Exit?"=w315:bool)
        n123 = Select(t="UI: Front Panel State >> Close", s=w315, f="") -> (s? t:f=w312:string)
        n124 = call <vilib>:"Add State(s) to Queue__jki_lib_state_machine.vi"("State(s) in (\"\")"=w312, "State(s) at Back (\"\")"="Connection: Close\nData: Cleanup\nExit") -> ("States Out"=w310:string)  [unwired: 13 in]
        n125 = call <vilib>:"Add State(s) to Queue__jki_lib_state_machine.vi"("State(s) in Front (\"\")"=w310, "State(s) in (\"\")"=w319) -> ("States Out"=w318:string)  [unwired: 13 in]
      }
      frame "---------- Manage ----------" {
        # "Template Separator\n(You can make a copy of, or modify, this frame)"
        n126 = call <vilib>:"Add State(s) to Queue__jki_lib_state_machine.vi"("State(s) in (\"\")"=w323) -> ("States Out"=w322:string)  [unwired: 14 in]
      }
      frame "Manage: Get Tables" {
        # "Your code here.\n(You can make a copy of, or modify, this frame)"
        n127 = Unbundle By Name(w330) -> ("Data.PG"=w328:refnum<class "LV-Data.PGSQL.lvclass">)
        n128 = call "List Tables.vi"("error in (no error)"=w326, "Data.PG"=w328) -> ("error out"=w325:errorcluster, "Table Paths"=w324:string[], "Table Names"=w327:string[])  [unwired: 6 in, 1 out]
        n129 = Bundle By Name(cluster=w330, "table names"=w327, "table paths"=w324) -> (w329:T4)
        n130 = call <vilib>:"Add State(s) to Queue__jki_lib_state_machine.vi"("State(s) in (\"\")"=w332) -> ("States Out"=w331:string)  [unwired: 14 in]
      }
      frame "Manage: Get Columns" {
        # "Your code here.\n(You can make a copy of, or modify, this frame)"
        n131 = Unbundle By Name(w343) -> ("Data.PG"=w340:refnum<class "LV-Data.PGSQL.lvclass">, "selected table path"=w339:string)
        n132 = call "List Columns.vi"("error in (no error)"=w338, "Table Path"=w339, "Data.PG"=w340) -> ("error out"=w337:errorcluster, "Column Paths"=w334:string[], "Column Names"=w336:string[], "Data.PG out"=w333:refnum<class "LV-Data.PGSQL.lvclass">, "Column Units"=w335:string[])  [unwired: 4 in]
        n133 = Bundle By Name(cluster=w343, "Data.PG"=w333, "column names"=w336, "column units"=w334, "column paths"=w335) -> (w342:T4)
        n134 = call <vilib>:"Add State(s) to Queue__jki_lib_state_machine.vi"("State(s) in Front (\"\")"="UI: Initialize" ("State(s) in Front (\"\")"), "State(s) in (\"\")"=w345) -> ("States Out"=w344:string)  [unwired: 13 in]
      }
      frame "Manage: Create Table" {
        # "Template Separator\n(You can make a copy of, or modify, this frame)"
        n135 = Unbundle By Name(w346) -> ("Data.PG"=w354:refnum<class "LV-Data.PGSQL.lvclass">, "table paths"=w350:string[], "new table name"=w347:string)
        n136 = call "Create Table.vi"("error in (no error)"=w349, "New Table Name"=w347, "Table Paths"=w350, "Data.PGSQL"=w354) -> ("error out"=w348:errorcluster, "Data.PGSQL out"=w351:refnum<class "LV-Data.PGSQL.lvclass">)  [unwired: 6 in]
        n137 = Bundle By Name(cluster=w346, "Data.PG"=w351) -> (w352:T4)
        n138 = call <vilib>:"Add State(s) to Queue__jki_lib_state_machine.vi"("State(s) in Front (\"\")"="Manage: Get Tables\nUI: Initialize" ("State(s) in Front (\"\")"), "State(s) in (\"\")"=w356) -> ("States Out"=w355:string)  [unwired: 13 in]
      }
      frame "Manage: Create Column" {
        # "Template Separator\n(You can make a copy of, or modify, this frame)"
        n139 = Unbundle By Name(w359) -> ("Data.PG"=w366:refnum<class "LV-Data.PGSQL.lvclass">, "selected table path"=w357:string, "new column data type"=w358:T1, "new column name"=w364:string, "new column units"=w363:string)
        n140 = call "Create Column.vi"("new column units"=w363, "Data type"=w358, "error in (no error)"=w365, "new column name"=w364, "selected table path"=w357, "Data.PGSQL in"=w366) -> ("error out"=w362:errorcluster, "Data.PGSQL out"=w360:refnum<class "LV-Data.PGSQL.lvclass">)  [unwired: 4 in]
        n141 = Bundle By Name(cluster=w359, "Data.PG"=w360) -> (w361:T4)
        n142 = call <vilib>:"Add State(s) to Queue__jki_lib_state_machine.vi"("State(s) in (\"\")"=w368) -> ("States Out"=w367:string)  [unwired: 14 in]
      }
      frame "Manage: Update Table Name" {
        # "Template Separator\n(You can make a copy of, or modify, this frame)"
        n143 = local read "New Table Name"() -> (w370:string)
        n144 = Unbundle By Name(w376) -> ("Data.PG"=w372:refnum<class "LV-Data.PGSQL.lvclass">, "selected table"=w369:string)
        n145 = call "Rename Table.vi"("error in"=w374, "New Table Name"=w370, "Existing Table Name"=w369, "Data.PG"=w372) -> ("error out"=w373:errorcluster, "Data.PG out"=w371:refnum<class "LV-Data.PGSQL.lvclass">)  [unwired: 5 in, 1 out]
        n146 = Bundle By Name(cluster=w376, "Data.PG"=w371) -> (w375:T4)
        n147 = call <vilib>:"Add State(s) to Queue__jki_lib_state_machine.vi"("State(s) in (\"\")"=w378) -> ("States Out"=w377:string)  [unwired: 14 in]
      }
      frame "Manage: Update Column Name" {
        # "Template Separator\n(You can make a copy of, or modify, this frame)"
        n148 = Unbundle By Name(w380) -> ("Data.PG"=w382:refnum<class "LV-Data.PGSQL.lvclass">, "selected table path"=w388:string, "selected column path"=w387:string)
        n149 = local read "New Column Name"() -> (w379:string)
        n150 = call "Change Column Name.vi"("New Column name"=w379, "error in (no error)"=w385, "selected column path"=w387, "selected table path"=w388, "Data.PGSQL in"=w382) -> ("error out"=w384:errorcluster, "Data.PGSQL out"=w381:refnum<class "LV-Data.PGSQL.lvclass">)  [unwired: 5 in]
        n151 = Bundle By Name(cluster=w380, "Data.PG"=w381, "selected column"=w379) -> (w383:T4)
        n152 = call <vilib>:"Add State(s) to Queue__jki_lib_state_machine.vi"("State(s) in Front (\"\")"="Manage: Get Columns\nUI: Choose Column\nData: Get Selected Column\nPaths: Get Column Path" ("State(s) in Front (\"\")"), "State(s) in (\"\")"=w390) -> ("States Out"=w389:string)  [unwired: 13 in]
      }
      frame "Manage: Update Column Units" {
        # "Template Separator\n(You can make a copy of, or modify, this frame)"
        n153 = Unbundle By Name(w398) -> ("Data.PG"=w396:refnum<class "LV-Data.PGSQL.lvclass">, "selected table path"=w397:string, "selected column path"=w393:string)
        n154 = local read "New Column Units"() -> (w391:string)
        n155 = call "Change Column Units.vi"("Change units"=w391, "error in (no error)"=w394, "selected column path"=w393, "selected table path"=w397, "Data.PG in"=w396) -> ("error out"=w392:errorcluster)  [unwired: 5 in, 1 out]
        n156 = call <vilib>:"Add State(s) to Queue__jki_lib_state_machine.vi"("State(s) in Front (\"\")"="Manage: Get Columns\nData: Get Selected Column\nPaths: Get Column Path" ("State(s) in Front (\"\")"), "State(s) in (\"\")"=w400) -> ("States Out"=w399:string)  [unwired: 13 in]
      }
      frame "Manage: Delete Column" {
        n157 = Unbundle By Name(w402) -> ("Data.PG"=w408:refnum<class "LV-Data.PGSQL.lvclass">, "selected table path"=w407:string, "selected column path"=w406:string)
        n158 = call "Delete Column.vi"("error in"=w404, "Column path"=w406, "Table Path"=w407, "LV-Data.PG"=w408) -> ("error out"=w403:errorcluster, "LV-Data.PG out"=w405:refnum<class "LV-Data.PGSQL.lvclass">)  [unwired: 6 in]
        n159 = Bundle By Name(cluster=w402, "Data.PG"=w405) -> (w401:T4)
        n160 = call <vilib>:"Add State(s) to Queue__jki_lib_state_machine.vi"("State(s) in (\"\")"=w409) -> ("States Out"=w410:string)  [unwired: 14 in]
      }
      frame "Manage: Delete Table" {
        n161 = Unbundle By Name(w412) -> ("Data.PG"=w417:refnum<class "LV-Data.PGSQL.lvclass">, "selected table path"=w416:string)
        n162 = call "Delete Table.vi"("error in"=w414, "Table Path"=w416, "LV-Data.PGSQL"=w417) -> ("error out"=w413:errorcluster, "LV-Data.PGSQL out"=w415:refnum<class "LV-Data.PGSQL.lvclass">)  [unwired: 7 in]
        n163 = Bundle By Name(cluster=w412, "Data.PG"=w415) -> (w411:T4)
        n164 = call <vilib>:"Add State(s) to Queue__jki_lib_state_machine.vi"("State(s) in (\"\")"=w418) -> ("States Out"=w419:string)  [unwired: 14 in]
      }
      frame "---------- Connection ----------" {
        # "Template Separator\n(You can make a copy of, or modify, this frame)"
        n165 = call <vilib>:"Add State(s) to Queue__jki_lib_state_machine.vi"("State(s) in (\"\")"=w423) -> ("States Out"=w422:string)  [unwired: 14 in]
      }
      frame "Connection: Open" {
        # "Template Separator\n(You can make a copy of, or modify, this frame)"
        n166 = Unbundle By Name(w428) -> ("Data.PG"=w426:refnum<class "LV-Data.PGSQL.lvclass">)
        n167 = call "PGSQL.Open.vi"("error in (no error)"=w425, "Data.PG in"=w426) -> ("error out"=w424:errorcluster, "Data.PG out"=w427:refnum<class "LV-Data.PGSQL.lvclass">)  [unwired: 8 in]
        n168 = Bundle By Name(cluster=w428, "Data.PG"=w427) -> (w429:T4)
        n169 = call <vilib>:"Add State(s) to Queue__jki_lib_state_machine.vi"("State(s) in (\"\")"=w431) -> ("States Out"=w430:string)  [unwired: 14 in]
      }
      frame "Connection: Close" {
        # "Template Separator\n(You can make a copy of, or modify, this frame)"
        n170 = Unbundle By Name(w435) -> ("Data.PG"=w434:refnum<class "LV-Data.PGSQL.lvclass">)
        n171 = call-dynamic "Close.vi"("error in (no error)"=w433, "Data.PG in"=w434) -> ("error out"=w432:errorcluster)  [unwired: 8 in, 1 out]
        n172 = call <vilib>:"Add State(s) to Queue__jki_lib_state_machine.vi"("State(s) in (\"\")"=w437) -> ("States Out"=w436:string)  [unwired: 14 in]
      }
      frame "---------- Paths ----------" {
        # "Template Separator\n(You can make a copy of, or modify, this frame)"
        n173 = call <vilib>:"Add State(s) to Queue__jki_lib_state_machine.vi"("State(s) in (\"\")"=w441) -> ("States Out"=w440:string)  [unwired: 14 in]
      }
      frame "Paths: Get Table Path" {
        # "Template Separator\n(You can make a copy of, or modify, this frame)"
        n174 = Unbundle By Name(w448) -> ("Data.PG"=w446:refnum<class "LV-Data.PGSQL.lvclass">, "selected table"=w445:string)
        n175 = call "Get Table Path.vi"("error in (no error)"=w444, "Table Name"=w445, "Data.PG"=w446) -> ("error out"=w443:errorcluster, "Table Path"=w442:string)  [unwired: 5 in, 2 out]
        n176 = Bundle By Name(cluster=w448, "selected table path"=w442) -> (w447:T4)
        n177 = call <vilib>:"Add State(s) to Queue__jki_lib_state_machine.vi"("State(s) in (\"\")"=w450) -> ("States Out"=w449:string)  [unwired: 14 in]
      }
      frame "Paths: Get Column Path" {
        # "Template Separator\n(You can make a copy of, or modify, this frame)"
        n178 = Unbundle By Name(w451) -> ("Data.PG"=w458:refnum<class "LV-Data.PGSQL.lvclass">, "selected table path"=w457:string, "selected column"=w452:string, "selected table"=w461:string, "selected column"=w460:string)
        n179 = call "Get Column Path.vi"("error in (no error)"=w456, "Column Name"=w452, "Table path"=w457, "Data.PG in"=w458) -> ("error out"=w453:errorcluster, "Column Unit"=w454:string, "Column Path"=w455:string)  [unwired: 4 in, 1 out]
        n180 = Bundle By Name(cluster=w451, "selected column path"=w455, "selected column units"=w454) -> (w464:T4)
        n181 = call "Build Path.vi"("Table path"=w457, "Column path"=w455, "Table name"=w461, "Column name"=w460, "Column units"=w454) -> ("PG path"=→"Path":string)  [unwired: 10 in]
        n182 = call <vilib>:"Add State(s) to Queue__jki_lib_state_machine.vi"("State(s) in (\"\")"=w462) -> ("States Out"=w463:string)  [unwired: 14 in]
      }
    }
  }
